vi "Handle Error.vi"(8 "Error In":errorcluster, 11 "Reader In":refnum<class "Reader.lvclass">) -> (0 "Error Out":errorcluster, 3 "Reader Out":refnum<class "Reader.lvclass">)   [LabVIEW 2018, in "Toolkit.lvlib" / "Reader.lvclass"]
uses:
  Reader.lvclass
  Reader.lvclass/Reader.ctl
  Toolkit.lvlib
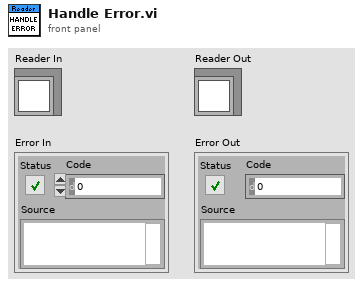
[diagram p1: front panel]
types:
  T1 = typedef "Toolkit.lvlib/Status.ctl" = enum32{"OK", "Out of Memory", "Null Value", "Encoder", "Decoder"}
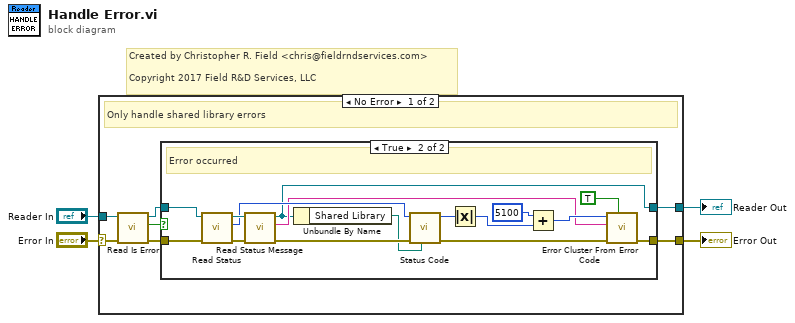
[diagram p0: block diagram]
diagram:
  # "Created by Christopher R. Field <chris@fieldrndservices.com>\n\nCopyright 2017 Field R&D Services, LLC"
  n1 = case shown="No Error" "Error In" {
    selector: "Error In" -> [w5 w30]
    tunnel: [w11 w31] -> w1
    tunnel: [w10 w30] -> w4
    tunnel: "Reader In" -> [w6 w31]
    frame No Error {
      # "Only handle shared library errors"
      n2 = call "Read Is Error.vi"("Error In"=w5, "Reader In"=w6) -> ("Error Out"=w9:errorcluster, "Error"=w7:bool, "Reader Out"=w8:refnum<class "Reader.lvclass">)  [unwired: 7 in]
      n3 = case shown="True" w7 {
        tunnel: w8 -> [w13 w28]
        tunnel: w9 -> [w12 w29]
        tunnel: [w12 w16] -> w10
        tunnel: [w13 w15] -> w11
        frame False {
          # "No Error"
        }
        frame True {
          # "Error occurred"
          n4 = call "Read Status.vi"("Error In"=w29, "Reader In"=w28) -> ("Error Out"=w27:errorcluster, "Status"=w24:T1, "Reader Out"=w26:refnum<class "Reader.lvclass">)  [unwired: 7 in]
          n5 = call "Read Status Message.vi"("Error In"=w27, "Reader In"=w26) -> ("Error Out"=w25:errorcluster, "Message"=w19:string, "Reader Out"=w15:refnum<class "Reader.lvclass">)  [unwired: 7 in]
          n6 = Unbundle By Name(w15) -> ("Shared Library"=w14:path)
          n7 = call "Status Code.vi"("LabPack Shared Library"=w14, "Error In"=w25, "Status"=w24) -> ("Error Out"=w17:errorcluster, "Code"=w22:i32)  [unwired: 7 in]
          n8 = Absolute Value(x=w22) -> (abs(x)=w21:i32)
          n9 = Add(x=5100, y=w21) -> (x+y=w20:i32)
          n10 = call <vilib>:"Error Cluster From Error Code.vi"("show call chain? (False)"=TRUE, "error in (no error)"=w17, "error message (\"\")"=w19, "error code (0)"=w20) -> ("error out"=w16:errorcluster)  [unwired: 5 in]
        }
      }
    }
    frame Error {
      # "Just pass along any LabVIEW errors"
    }
  }
  "Error Out" <- w4
  "Reader Out" <- w1
